vi "SrReplaceByOffsetAndLength.vi"(8 "Replace":string[](array[string]), 9 "Lengths":i32[](array[numeric]), 10 "Offsets":i32[](array[numeric]), 11 "String":string) -> (3 "String":string)   [LabVIEW 2021, in "libpcre2-8.lvlib"]
uses:
  libpcre2-8.lvlib
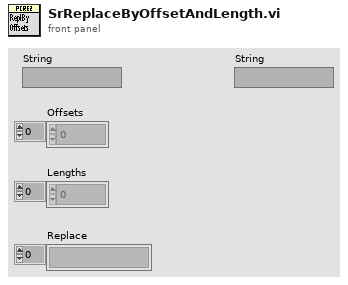
[diagram p1: front panel]
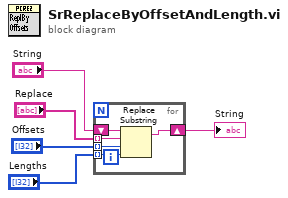
[diagram p0: block diagram]
diagram:
  n1 = for {
    tunnel: "Offsets" -> [w9] mode=indexing
    tunnel: "Lengths" -> [w8] mode=indexing
    tunnel: "Replace" -> [w7] mode=indexing
    shift-right: [w6] -> w4
    shift-left: "String" -> [w10]
    n2 = Replace Substring(2:w8, 3:w9, 4:w7, 5:w10) -> (1:w6:string)  [unwired: 1 out]
  }
  "String" <- w4
